vi "采集频点值.vi"(2 "频率点（MHZ）":string[](array[string])=["100", "1000", "2080", "3000", "5000", "6000"], 3 "测试对名称":string[](array[string])=["TX1", "RX1", "TX2", "RX2", "TX3", "RX3", "TX4", "RX4"], 4 "S参数测试项目":string[](array[string])=["SDD21", "SDD11", "SCD21", "SCD11"], 5 "TXT文件所处路径":path=path "C:/Users/wmg/Desktop/TXT") -> (0 "测试项目及频点在DB输出":string="$SDD21 TX1 100MHZ -0.86037 1000MHZ -3.12043 2080MHZ -4.75217 3000MHZ -5.83246 5000MHZ -8.12344 6000MHZ -9.17913:           RX1 100MHZ -0.81938 1000MHZ -3.13617 2080MHZ -4.81920 3000MHZ -6.02219 5000MHZ -8.41771 6000MHZ -9.33927:           TX2 100MHZ -0.85378 1000MHZ -3.08573 2080MHZ -4.67016 3000MHZ -5.78195 5000MHZ -8.32928 6000MHZ -9.19630:           RX2 100MHZ -0.86254 1000MHZ -3.12635 2080MHZ -4.75196 3000MHZ -5.88385 5000MHZ -8.13036 6000MHZ -9.13235:           TX3 100MHZ -0.86849 1000MHZ -3.14410 2080MHZ -4.79978 3000MHZ -5.90907 5000MHZ -8.13990 6000MHZ -9.11839:           RX3 100MHZ -0.86098 1000MHZ -3.12214 2080MHZ -4.73963 3000MHZ -5.88060 5000MHZ -8.20582 6000MHZ -9.38458:           TX4 100MHZ -0.86089 1000MHZ -3.13176 2080MHZ -4.75236 3000MHZ -5.88669 5000MHZ -8.11560 6000MHZ -9.08824:           RX4 100MHZ -0.86019 1000MHZ -3.12295 2080MHZ -4.74843 3000MHZ -5.87279 5000MHZ -8.16658 6000MHZ -9.27592#:SDD11 TX1 100MHZ -0.86037 1000MHZ -3.12043 2080MHZ -4.75217 3000MHZ -5.83246 5000MHZ -8.12344 6000MHZ -9.17913:           RX1 100MHZ -0.81938 1000MHZ -3.13617 2080MHZ -4.81920 3000MHZ -6.02219 5000MHZ -8.41771 6000MHZ -9.33927:           TX2 100MHZ -0.85378 1000MHZ -3.08573 2080MHZ -4.67016 3000MHZ -5.78195 5000MHZ -8.32928 6000MHZ -9.19630:           RX2 100MHZ -0.86254 1000MHZ -3.12635 2080MHZ -4.75196 3000MHZ -5.88385 5000MHZ -8.13036 6000MHZ -9.13235:           TX3 100MHZ -0.86849 1000MHZ -3.14410 2080MHZ -4.79978 3000MHZ -5.90907 5000MHZ -8.13990 6000MHZ -9.11839:           RX3 100MHZ -0.86098 1000MHZ -3.12214 2080MHZ -4.73963 3000MHZ -5.88060 5000MHZ -8.20582 6000MHZ -9.38458:           TX4 100MHZ -0.86089 1000MHZ -3.13176 2080MHZ -4.75236 3000MHZ -5.88669 5000MHZ -8.11560 6000MHZ -9.08824:           RX4 100MHZ -0.86019 1000MHZ -3.12295 2080MHZ -4.74843 3000MHZ -5.87279 5000MHZ -8.16658 6000MHZ -9.27592#:SCD21 TX1 100MHZ -0.86037 1000MHZ -3.12043 2080MHZ -4.75217 3000MHZ -5.83246 5000MHZ -8.12344 6000MHZ -9.17913:           RX1 100MHZ -0.81938 1000MHZ -3.13617 2080MHZ -4.81920 3000MHZ -6.02219 5000MHZ -8.41771 6000MHZ -9.33927:           TX2 100MHZ -0.85378 1000MHZ -3.08573 2080MHZ -4.67016 3000MHZ -5.78195 5000MHZ -8.32928 6000MHZ -9.19630:           RX2 100MHZ -0.86254 1000MHZ -3.12635 2080MHZ -4.75196 3000MHZ -5.88385 5000MHZ -8.13036 6000MHZ -9.13235:           TX3 100MHZ -0.86849 1000MHZ -3.14410 2080MHZ -4.79978 3000MHZ -5.90907 5000MHZ -8.13990 6000MHZ -9.11839:           RX3 100MHZ -0.86098 1000MHZ -3.12214 2080MHZ -4.73963 3000MHZ -5.88060 5000MHZ -8.20582 6000MHZ -9.38458:           TX4 100MHZ -0.86089 1000MHZ -3.13176 2080MHZ -4.75236 3000MHZ -5.88669 5000MHZ -8.11560 6000MHZ -9.08824:           RX4 100MHZ -0.86019 1000MHZ -3.12295 2080MHZ -4.74843 3000MHZ -5.87279 5000MHZ -8.16658 6000MHZ -9.27592#:SCD11 TX1 100MHZ -0.86037 1000MHZ -3.12043 2080MHZ -4.75217 3000MHZ -5.83246 5000MHZ -8.12344 6000MHZ -9.17913:           RX1 100MHZ -0.81938 1000MHZ -3.13617 2080MHZ -4.81920 3000MHZ -6.02219 5000MHZ -8.41771 6000MHZ -9.33927:           TX2 100MHZ -0.85378 1000MHZ -3.08573 2080MHZ -4.67016 3000MHZ -5.78195 5000MHZ -8.32928 6000MHZ -9.19630:           RX2 100MHZ -0.86254 1000MHZ -3.12635 2080MHZ -4.75196 3000MHZ -5.88385 5000MHZ -8.13036 6000MHZ -9.13235:           TX3 100MHZ -0.86849 1000MHZ -3.14410 2080MHZ -4.79978 3000MHZ -5.90907 5000MHZ -8.13990 6000MHZ -9.11839:           RX3 100MHZ -0.86098 1000MHZ -3.12214 2080MHZ -4.73963 3000MHZ -5.88060 5000MHZ -8.20582 6000MHZ -9.38458:           TX4 100MHZ -0.86089 1000MHZ -3.13176 2080MHZ -4.75236 3000MHZ -5.88669 5000MHZ -8.11560 6000MHZ -9.08824:           RX4 100MHZ -0.86019 1000MHZ -3.12295 2080MHZ -4.74843 3000MHZ -5.87279 5000MHZ -8.16658 6000MHZ -9.27592#$", 1 "测试项目及频点在txt输出":string="$\nSDD21 TX1 100MHZ -0.86037 1000MHZ -3.12043 2080MHZ -4.75217 3000MHZ -5.83246 5000MHZ -8.12344 6000MHZ -9.17913\n           RX1 100MHZ -0.81938 1000MHZ -3.13617 2080MHZ -4.81920 3000MHZ -6.02219 5000MHZ -8.41771 6000MHZ -9.33927\n           TX2 100MHZ -0.85378 1000MHZ -3.08573 2080MHZ -4.67016 3000MHZ -5.78195 5000MHZ -8.32928 6000MHZ -9.19630\n           RX2 100MHZ -0.86254 1000MHZ -3.12635 2080MHZ -4.75196 3000MHZ -5.88385 5000MHZ -8.13036 6000MHZ -9.13235\n           TX3 100MHZ -0.86849 1000MHZ -3.14410 2080MHZ -4.79978 3000MHZ -5.90907 5000MHZ -8.13990 6000MHZ -9.11839\n           RX3 100MHZ -0.86098 1000MHZ -3.12214 2080MHZ -4.73963 3000MHZ -5.88060 5000MHZ -8.20582 6000MHZ -9.38458\n           TX4 100MHZ -0.86089 1000MHZ -3.13176 2080MHZ -4.75236 3000MHZ -5.88669 5000MHZ -8.11560 6000MHZ -9.08824\n           RX4 100MHZ -0.86019 1000MHZ -3.12295 2080MHZ -4.74843 3000MHZ -5.87279 5000MHZ -8.16658 6000MHZ -9.27592#\nSDD11 TX1 100MHZ -0.86037 1000MHZ -3.12043 2080MHZ -4.75217 3000MHZ -5.83246 5000MHZ -8.12344 6000MHZ -9.17913\n           RX1 100MHZ -0.81938 1000MHZ -3.13617 2080MHZ -4.81920 3000MHZ -6.02219 5000MHZ -8.41771 6000MHZ -9.33927\n           TX2 100MHZ -0.85378 1000MHZ -3.08573 2080MHZ -4.67016 3000MHZ -5.78195 5000MHZ -8.32928 6000MHZ -9.19630\n           RX2 100MHZ -0.86254 1000MHZ -3.12635 2080MHZ -4.75196 3000MHZ -5.88385 5000MHZ -8.13036 6000MHZ -9.13235\n           TX3 100MHZ -0.86849 1000MHZ -3.14410 2080MHZ -4.79978 3000MHZ -5.90907 5000MHZ -8.13990 6000MHZ -9.11839\n           RX3 100MHZ -0.86098 1000MHZ -3.12214 2080MHZ -4.73963 3000MHZ -5.88060 5000MHZ -8.20582 6000MHZ -9.38458\n           TX4 100MHZ -0.86089 1000MHZ -3.13176 2080MHZ -4.75236 3000MHZ -5.88669 5000MHZ -8.11560 6000MHZ -9.08824\n           RX4 100MHZ -0.86019 1000MHZ -3.12295 2080MHZ -4.74843 3000MHZ -5.87279 5000MHZ -8.16658 6000MHZ -9.27592#\nSCD21 TX1 100MHZ -0.86037 1000MHZ -3.12043 2080MHZ -4.75217 3000MHZ -5.83246 5000MHZ -8.12344 6000MHZ -9.17913\n           RX1 100MHZ -0.81938 1000MHZ -3.13617 2080MHZ -4.81920 3000MHZ -6.02219 5000MHZ -8.41771 6000MHZ -9.33927\n           TX2 100MHZ -0.85378 1000MHZ -3.08573 2080MHZ -4.67016 3000MHZ -5.78195 5000MHZ -8.32928 6000MHZ -9.19630\n           RX2 100MHZ -0.86254 1000MHZ -3.12635 2080MHZ -4.75196 3000MHZ -5.88385 5000MHZ -8.13036 6000MHZ -9.13235\n           TX3 100MHZ -0.86849 1000MHZ -3.14410 2080MHZ -4.79978 3000MHZ -5.90907 5000MHZ -8.13990 6000MHZ -9.11839\n           RX3 100MHZ -0.86098 1000MHZ -3.12214 2080MHZ -4.73963 3000MHZ -5.88060 5000MHZ -8.20582 6000MHZ -9.38458\n           TX4 100MHZ -0.86089 1000MHZ -3.13176 2080MHZ -4.75236 3000MHZ -5.88669 5000MHZ -8.11560 6000MHZ -9.08824\n           RX4 100MHZ -0.86019 1000MHZ -3.12295 2080MHZ -4.74843 3000MHZ -5.87279 5000MHZ -8.16658 6000MHZ -9.27592#\nSCD11 TX1 100MHZ -0.86037 1000MHZ -3.12043 2080MHZ -4.75217 3000MHZ -5.83246 5000MHZ -8.12344 6000MHZ -9.17913\n           RX1 100MHZ -0.81938 1000MHZ -3.13617 2080MHZ -4.81920 3000MHZ -6.02219 5000MHZ -8.41771 6000MHZ -9.33927\n           TX2 100MHZ -0.85378 1000MHZ -3.08573 2080MHZ -4.67016 3000MHZ -5.78195 5000MHZ -8.32928 6000MHZ -9.19630\n           RX2 100MHZ -0.86254 1000MHZ -3.12635 2080MHZ -4.75196 3000MHZ -5.88385 5000MHZ -8.13036 6000MHZ -9.13235\n           TX3 100MHZ -0.86849 1000MHZ -3.14410 2080MHZ -4.79978 3000MHZ -5.90907 5000MHZ -8.13990 6000MHZ -9.11839\n           RX3 100MHZ -0.86098 1000MHZ -3.12214 2080MHZ -4.73963 3000MHZ -5.88060 5000MHZ -8.20582 6000MHZ -9.38458\n           TX4 100MHZ -0.86089 1000MHZ -3.13176 2080MHZ -4.75236 3000MHZ -5.88669 5000MHZ -8.11560 6000MHZ -9.08824\n           RX4 100MHZ -0.86019 1000MHZ -3.12295 2080MHZ -4.74843 3000MHZ -5.87279 5000MHZ -8.16658 6000MHZ -9.27592#$\n")   [LabVIEW 2011]
uses:
  <vilib>/Utility/file.llb/Read From Spreadsheet File (string).vi
panel:
  out "数组 2":string[](array[string])=["SDD21 TX1 100MHZ -0.86037 1000MHZ -3.12043 2080MHZ -4.75217 3000MHZ -5.83246 5000MHZ -8.12344 6000MHZ -9.17913\n           RX1 100MHZ -0.81938 1000MHZ -3.13617 2080MHZ -4.81920 3000MHZ -6.02219 5000MHZ -8.41771 6000MHZ -9.33927\n           TX2 100MHZ -0.85378 1000MHZ -3.08573 2080MHZ -4.67016 3000MHZ -5.78195 5000MHZ -8.32928 6000MHZ -9.19630\n           RX2 100MHZ -0.86254 1000MHZ -3.12635 2080MHZ -4.75196 3000MHZ -5.88385 5000MHZ -8.13036 6000MHZ -9.13235\n           TX3 100MHZ -0.86849 1000MHZ -3.14410 2080MHZ -4.79978 3000MHZ -5.90907 5000MHZ -8.13990 6000MHZ -9.11839\n           RX3 100MHZ -0.86098 1000MHZ -3.12214 2080MHZ -4.73963 3000MHZ -5.88060 5000MHZ -8.20582 6000MHZ -9.38458\n           TX4 100MHZ -0.86089 1000MHZ -3.13176 2080MHZ -4.75236 3000MHZ -5.88669 5000MHZ -8.11560 6000MHZ -9.08824\n           RX4 100MHZ -0.86019 1000MHZ -3.12295 2080MHZ -4.74843 3000MHZ -5.87279 5000MHZ -8.16658 6000MHZ -9.27592#", "SDD11 TX1 100MHZ -0.86037 1000MHZ -3.12043 2080MHZ -4.75217 3000MHZ -5.83246 5000MHZ -8.12344 6000MHZ -9.17913\n           RX1 100MHZ -0.81938 1000MHZ -3.13617 2080MHZ -4.81920 3000MHZ -6.02219 5000MHZ -8.41771 6000MHZ -9.33927\n           TX2 100MHZ -0.85378 1000MHZ -3.08573 2080MHZ -4.67016 3000MHZ -5.78195 5000MHZ -8.32928 6000MHZ -9.19630\n           RX2 100MHZ -0.86254 1000MHZ -3.12635 2080MHZ -4.75196 3000MHZ -5.88385 5000MHZ -8.13036 6000MHZ -9.13235\n           TX3 100MHZ -0.86849 1000MHZ -3.14410 2080MHZ -4.79978 3000MHZ -5.90907 5000MHZ -8.13990 6000MHZ -9.11839\n           RX3 100MHZ -0.86098 1000MHZ -3.12214 2080MHZ -4.73963 3000MHZ -5.88060 5000MHZ -8.20582 6000MHZ -9.38458\n           TX4 100MHZ -0.86089 1000MHZ -3.13176 2080MHZ -4.75236 3000MHZ -5.88669 5000MHZ -8.11560 6000MHZ -9.08824\n           RX4 100MHZ -0.86019 1000MHZ -3.12295 2080MHZ -4.74843 3000MHZ -5.87279 5000MHZ -8.16658 6000MHZ -9.27592#", "SCD21 TX1 100MHZ -0.86037 1000MHZ -3.12043 2080MHZ -4.75217 3000MHZ -5.83246 5000MHZ -8.12344 6000MHZ -9.17913\n           RX1 100MHZ -0.81938 1000MHZ -3.13617 2080MHZ -4.81920 3000MHZ -6.02219 5000MHZ -8.41771 6000MHZ -9.33927\n           TX2 100MHZ -0.85378 1000MHZ -3.08573 2080MHZ -4.67016 3000MHZ -5.78195 5000MHZ -8.32928 6000MHZ -9.19630\n           RX2 100MHZ -0.86254 1000MHZ -3.12635 2080MHZ -4.75196 3000MHZ -5.88385 5000MHZ -8.13036 6000MHZ -9.13235\n           TX3 100MHZ -0.86849 1000MHZ -3.14410 2080MHZ -4.79978 3000MHZ -5.90907 5000MHZ -8.13990 6000MHZ -9.11839\n           RX3 100MHZ -0.86098 1000MHZ -3.12214 2080MHZ -4.73963 3000MHZ -5.88060 5000MHZ -8.20582 6000MHZ -9.38458\n           TX4 100MHZ -0.86089 1000MHZ -3.13176 2080MHZ -4.75236 3000MHZ -5.88669 5000MHZ -8.11560 6000MHZ -9.08824\n           RX4 100MHZ -0.86019 1000MHZ -3.12295 2080MHZ -4.74843 3000MHZ -5.87279 5000MHZ -8.16658 6000MHZ -9.27592#", "SCD11 TX1 100MHZ -0.86037 1000MHZ -3.12043 2080MHZ -4.75217 3000MHZ -5.83246 5000MHZ -8.12344 6000MHZ -9.17913\n           RX1 100MHZ -0.81938 1000MHZ -3.13617 2080MHZ -4.81920 3000MHZ -6.02219 5000MHZ -8.41771 6000MHZ -9.33927\n           TX2 100MHZ -0.85378 1000MHZ -3.08573 2080MHZ -4.67016 3000MHZ -5.78195 5000MHZ -8.32928 6000MHZ -9.19630\n           RX2 100MHZ -0.86254 1000MHZ -3.12635 2080MHZ -4.75196 3000MHZ -5.88385 5000MHZ -8.13036 6000MHZ -9.13235\n           TX3 100MHZ -0.86849 1000MHZ -3.14410 2080MHZ -4.79978 3000MHZ -5.90907 5000MHZ -8.13990 6000MHZ -9.11839\n           RX3 100MHZ -0.86098 1000MHZ -3.12214 2080MHZ -4.73963 3000MHZ -5.88060 5000MHZ -8.20582 6000MHZ -9.38458\n           TX4 100MHZ -0.86089 1000MHZ -3.13176 2080MHZ -4.75236 3000MHZ -5.88669 5000MHZ -8.11560 6000MHZ -9.08824\n           RX4 100MHZ -0.86019 1000MHZ -3.12295 2080MHZ -4.74843 3000MHZ -5.87279 5000MHZ -8.16658 6000MHZ -9.27592#"]
  # "1. MHZ改为实际数值\n    10MHZ写为 10 000000\n2.冒号后面的空格去掉"
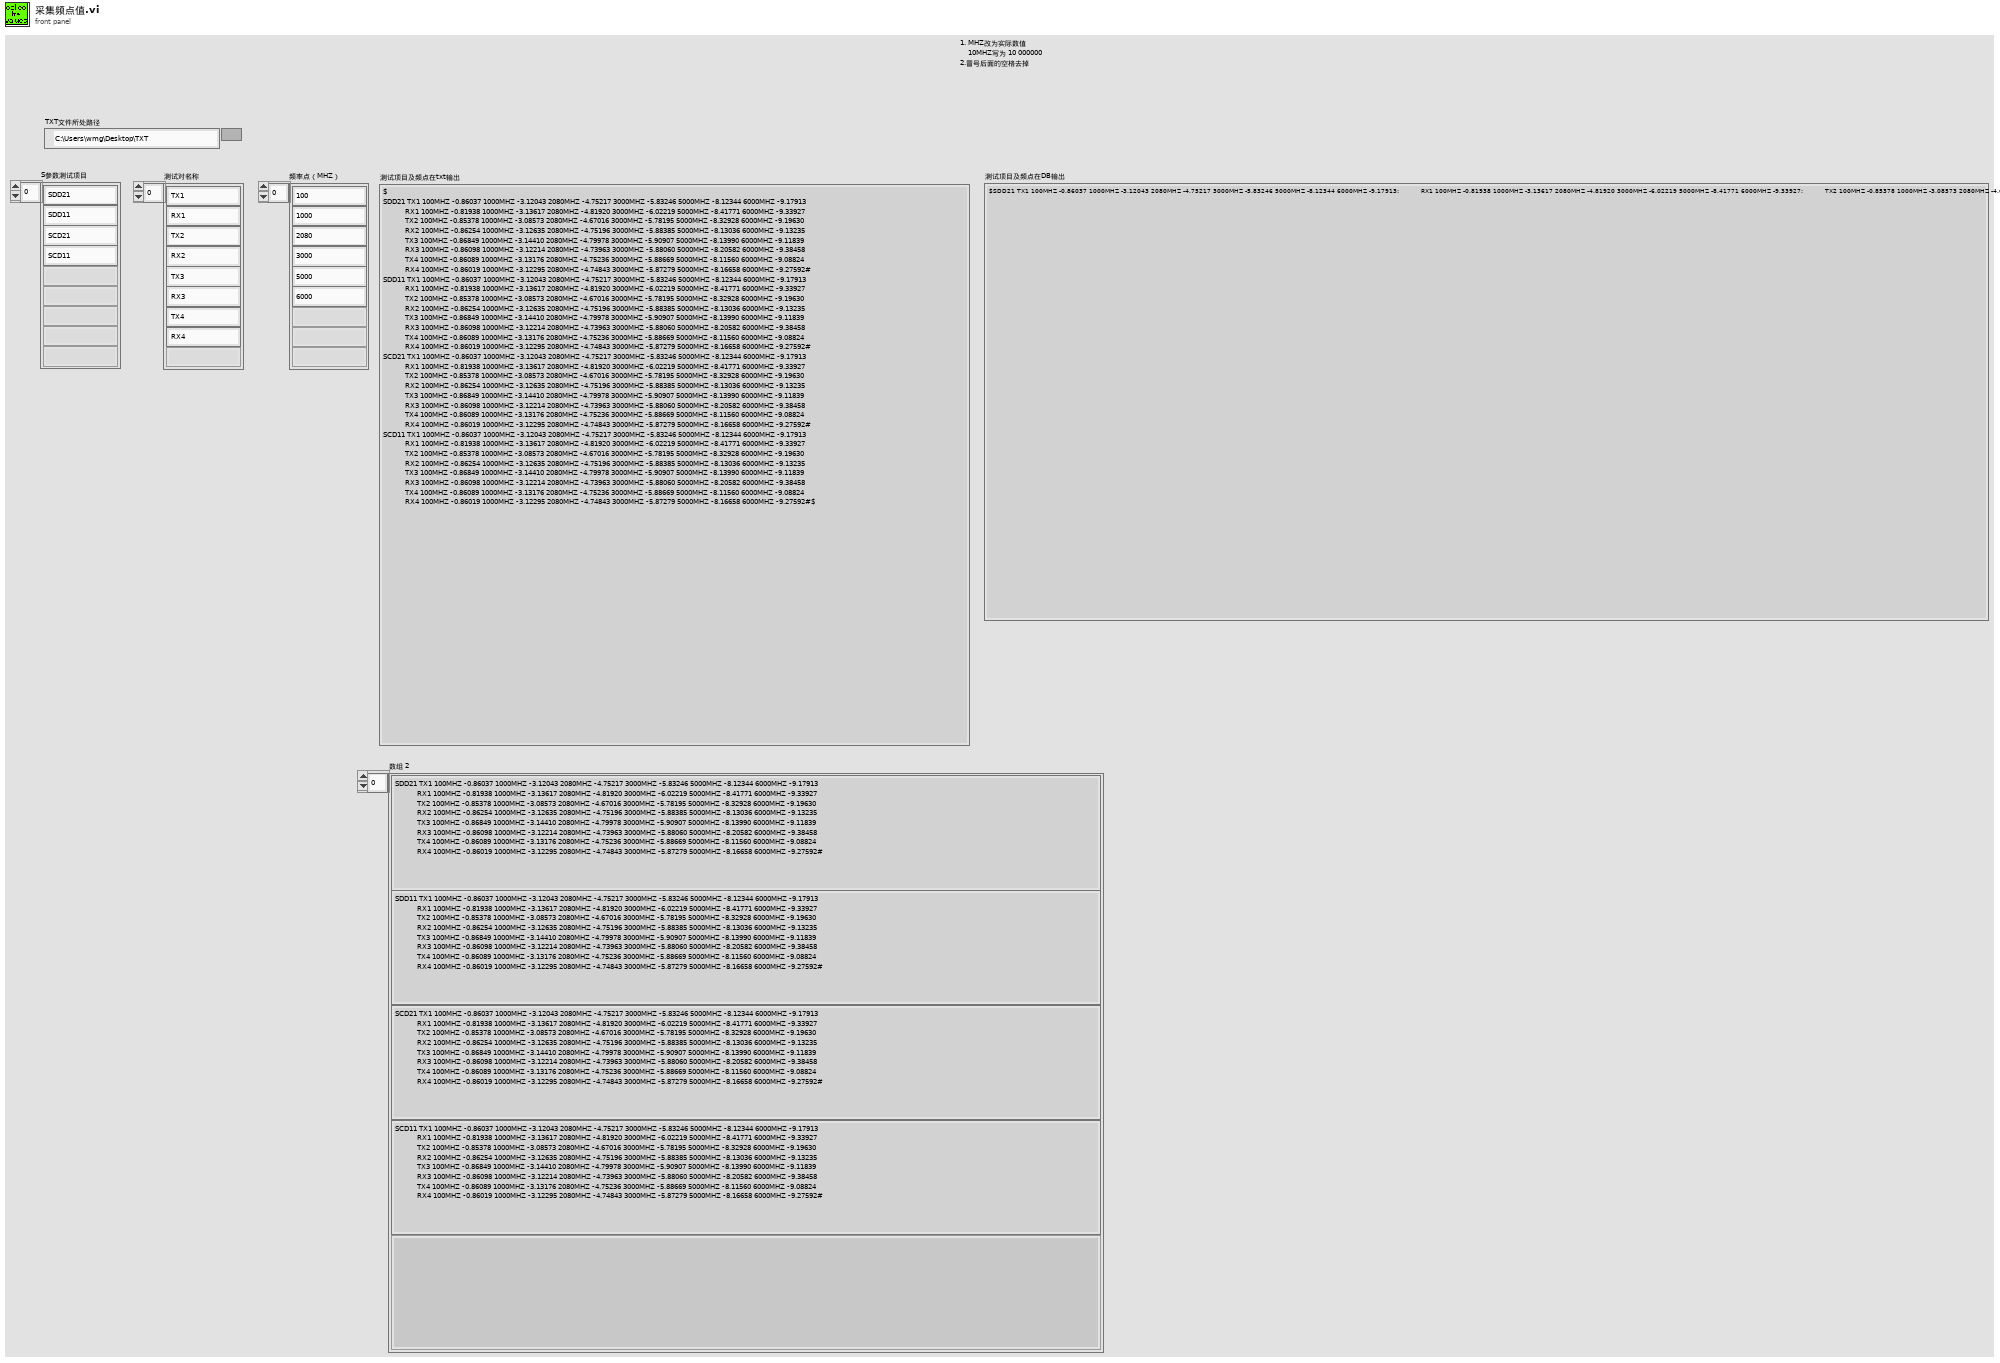
[diagram p1: front panel]
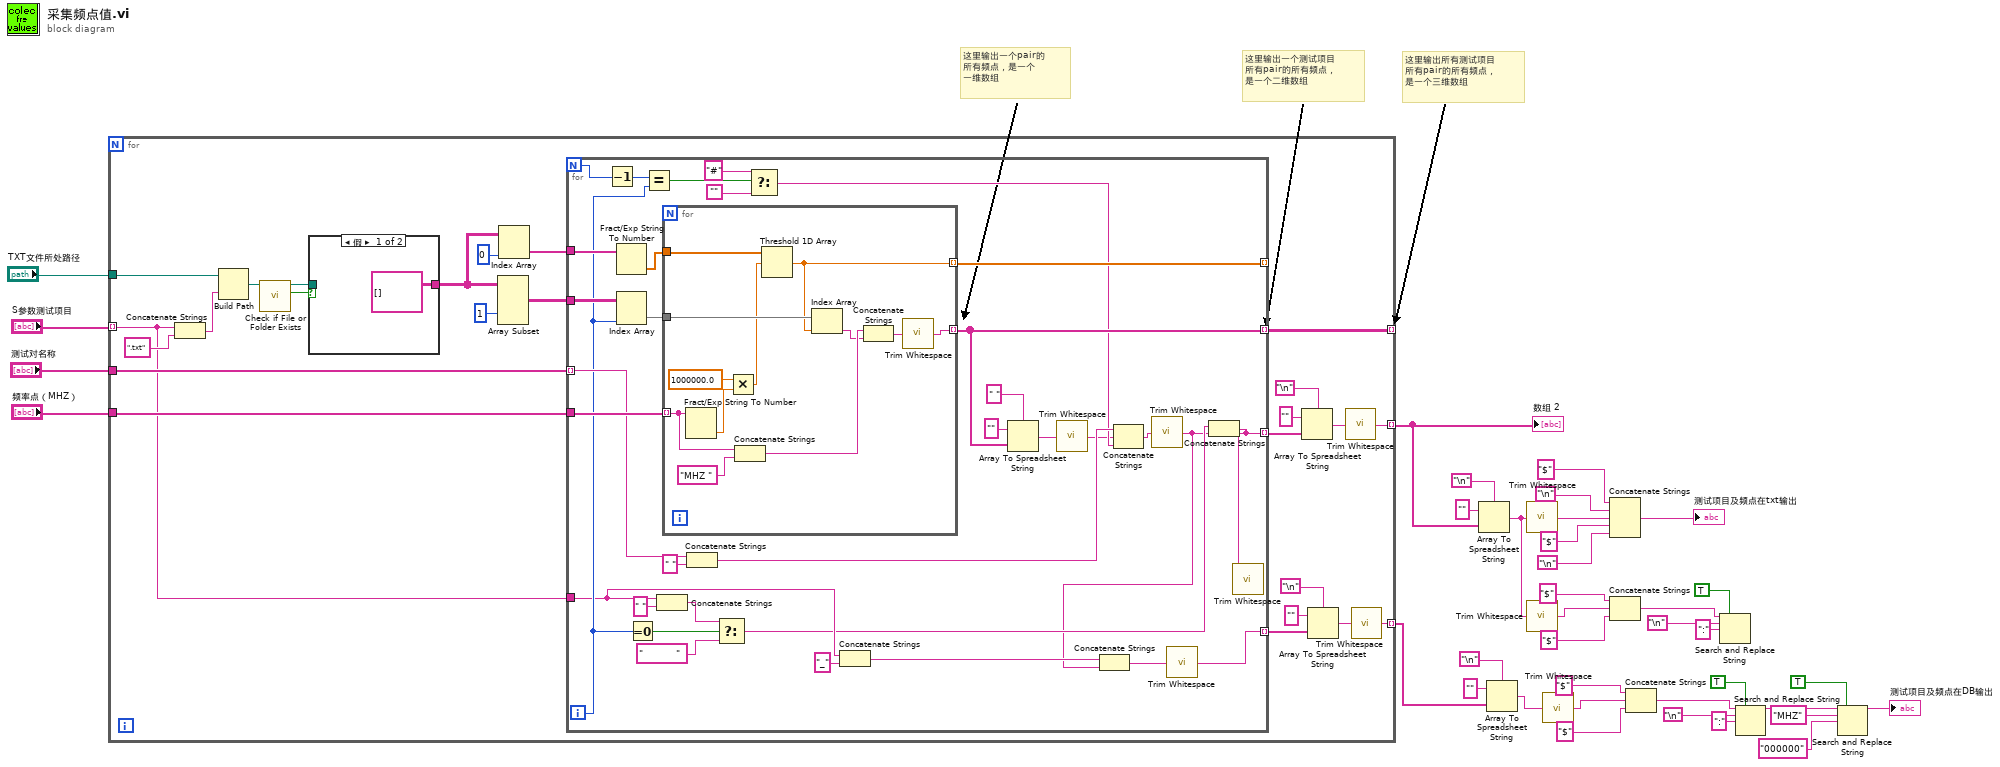
[diagram p0: block diagram]
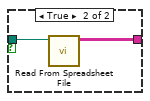
[diagram p2: hidden frame]
diagram:
  # "这里输出所有测试项目\n所有pair的所有频点，\n是一个三维数组"
  # "这里输出一个测试项目\n所有pair的所有频点，\n是一个二维数组"
  # "这里输出一个pair的\n所有频点，是一个\n一维数组"
  n1 = for {
    tunnel: "S参数测试项目" -> [w47] mode=indexing
    tunnel: "测试对名称" -> [w57]
    tunnel: "频率点（MHZ）" -> [w56]
    tunnel: "TXT文件所处路径" -> [w62]
    tunnel: [w52] -> _ mode=indexing
    tunnel: [w46] -> w31 mode=indexing
    tunnel: [w38] -> w14 mode=indexing
    n2 = Concatenate Strings(w47, ".txt" ("字符串")) -> (w60:string)
    n3 = Build Path(base path=w62, name or relative path=w60) -> (appended path=w45:path)
    n4 = call <vilib>:"Check if File or Folder Exists.vi"("path"=w45) -> ("file or folder exists?"=w44:bool, "dup path"=w43:path)  [unwired: 8 in, 1 out]
    n5 = case shown="假" w44 {
      tunnel: [string[][] [] ("all rows") w65] -> w55
      tunnel: w43 -> [_ w64]
      frame False {
      }
      frame True {
        n6 = call-poly <vilib>:"Read From Spreadsheet File.vi"("file path (dialog if empty)"=w64) -> ("all rows"=w65:string[][])  [unwired: 6 in, 4 out]
      }
    }
    n7 = Array Subset(array=w55, index (col)=1 ("索引")) -> (w58:string[][])  [unwired: 3 in]
    n8 = Index Array(array=w55, index (col)=0 ("禁用的索引 (列)")) -> (element=w53:string[])  [unwired: 1 in]
    n9 = for {
      N -> [w81]
      tunnel: w58 -> [w99]
      tunnel: w57 -> [w90] mode=indexing
      tunnel: w56 -> [w98]
      tunnel: w53 -> [w97]
      tunnel: [w93] -> w52 mode=indexing
      tunnel: [w94] -> _ mode=indexing
      tunnel: [w73] -> w50 mode=indexing
      tunnel: w47 -> [w71]
      tunnel: [w68] -> w39 mode=indexing
      i -> [w79]
      n10 = Decrement(x=w81) -> (x-1=w80:i32)
      n11 = Fract/Exp String To Number(string=w97) -> (number=w96:dbl[])  [unwired: 3 in, 1 out]
      n12 = Index Array(array=w99, index (col)=w79) -> (element=w95:string[])  [unwired: 1 in]
      n13 = Equal To 0?(x=w79) -> (x = 0?=w85:bool)
      n14 = Equal?(x=w80, y=w79) -> (x = y?=w78:bool)
      n15 = Concatenate Strings(w71, " " ("字符串")) -> (w82:string)
      n16 = for {
        tunnel: w98 -> [w105] mode=indexing
        tunnel: w96 -> [w111]
        tunnel: w95 -> [w110]
        tunnel: [w100] -> w93 mode=indexing
        tunnel: [w109] -> w94 mode=indexing
        n17 = Fract/Exp String To Number(string=w105) -> (number=w108:dbl)  [unwired: 3 in, 1 out]
        n18 = Multiply(x=1000000.0, y=w108) -> (x*y=w107:dbl)
        n19 = Concatenate Strings(w105, "MHZ ") -> (w102:string)
        n20 = Threshold 1D Array(2:w107, 3:w111) -> (0:w109:dbl)  [unwired: 1 in]
        n21 = Index Array(array=w110, index=w109) -> (element=w101:string)
        n22 = Concatenate Strings(w102, w101) -> (w103:string)
        n23 = call <vilib>:"Trim Whitespace.vi"("string"=w103) -> ("trimmed string"=w100:string)  [unwired: 1 in]
      }
      n24 = Concatenate Strings(w90, " " ("字符串")) -> (w86:string)
      n25 = Select(t=w82, s=w85, f="           " ("字符串")) -> (s? t:f=w67:string)
      n26 = Select(t="#", s=w78, f="") -> (s? t:f=w75:string)
      n27 = Concatenate Strings(w71, "_" ("字符串")) -> (w70:string)
      n28 = Array To Spreadsheet String(delimiter (Tab)=" " ("分隔符(Tab)"), array=w93, 3:"" ("格式字符串")) -> (spreadsheet string=w88:string)
      n29 = call <vilib>:"Trim Whitespace.vi"("string"=w88) -> ("trimmed string"=w74:string)  [unwired: 1 in]
      n30 = Concatenate Strings(w86, w74, w75) -> (w87:string)
      n31 = call <vilib>:"Trim Whitespace.vi"("string"=w87) -> ("trimmed string"=w66:string)  [unwired: 1 in]
      n32 = Concatenate Strings(w70, w66) -> (w69:string)
      n33 = call <vilib>:"Trim Whitespace.vi"("string"=w69) -> ("trimmed string"=w68:string)  [unwired: 1 in]
      n34 = Concatenate Strings(w67, w66) -> (w73:string)
      n35 = call <vilib>:"Trim Whitespace.vi"("string"=w73) -> ()  [unwired: 1 in, 1 out]
    }
    n36 = Array To Spreadsheet String(delimiter (Tab)="\n", array=w50, 3:"" ("格式字符串")) -> (spreadsheet string=w49:string)
    n37 = Array To Spreadsheet String(delimiter (Tab)="\n", array=w39, 3:"" ("格式字符串")) -> (spreadsheet string=w41:string)
    n38 = call <vilib>:"Trim Whitespace.vi"("string"=w49) -> ("trimmed string"=w46:string)  [unwired: 1 in]
    n39 = call <vilib>:"Trim Whitespace.vi"("string"=w41) -> ("trimmed string"=w38:string)  [unwired: 1 in]
  }
  "数组 2" <- w31
  n40 = Array To Spreadsheet String(delimiter (Tab)="\n", array=w31, 3:"" ("格式字符串")) -> (spreadsheet string=w18:string)
  n41 = Array To Spreadsheet String(delimiter (Tab)="\n", array=w14, 3:"" ("格式字符串")) -> (spreadsheet string=w6:string)
  n42 = call <vilib>:"Trim Whitespace.vi"("string"=w18) -> ("trimmed string"=w30:string)  [unwired: 1 in]
  n43 = call <vilib>:"Trim Whitespace.vi"("string"=w18) -> ("trimmed string"=w19:string)  [unwired: 1 in]
  n44 = call <vilib>:"Trim Whitespace.vi"("string"=w6) -> ("trimmed string"=w12:string)  [unwired: 1 in]
  n45 = Concatenate Strings("$", "\n", w30, "$", "\n") -> (→"测试项目及频点在txt输出":string)
  n46 = Concatenate Strings("$", w19, "$") -> (w17:string)
  n47 = Concatenate Strings("$", w12, "$") -> (w13:string)
  n48 = Search and Replace String(replace all?=TRUE ("替换全部？(F)"), input string=w17, search string="\n", replace string=":" ("替换字符串(\"\")")) -> ()  [unwired: 4 in, 4 out]
  n49 = Search and Replace String(replace all?=TRUE ("替换全部？(F)"), input string=w13, search string="\n", replace string=":" ("替换字符串(\"\")")) -> (result string=w5:string)  [unwired: 4 in, 3 out]
  n50 = Search and Replace String(replace all?=TRUE ("替换全部？(F)"), input string=w5, search string="MHZ" ("搜索字符串"), replace string="000000" ("替换字符串(\"\")")) -> (result string=→"测试项目及频点在DB输出":string)  [unwired: 4 in, 3 out]
